vi "get_price.vi"(8 "error in (no error)":errorcluster, 11 "Furniture in":refnum<class "Furniture.lvclass">) -> (0 "error out":errorcluster, 2 "price":dbl, 3 "Furniture out":refnum<class "Furniture.lvclass">)   [LabVIEW 2024, in "Furniture.lvclass"]
uses:
  Furniture.lvclass
  Furniture.lvclass/Furniture.ctl
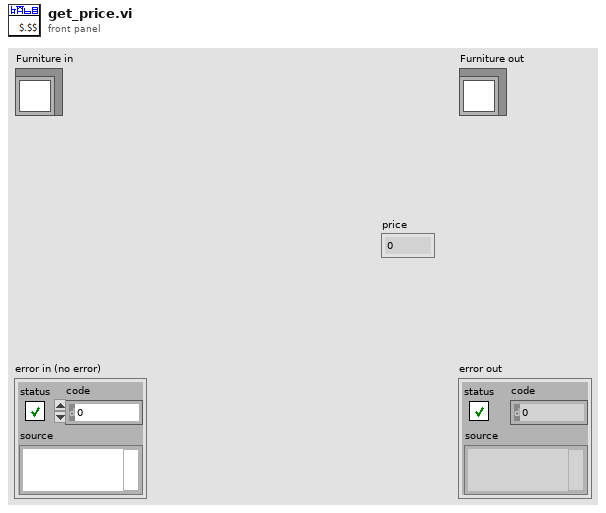
[diagram p1: front panel]
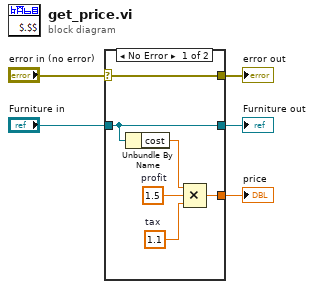
[diagram p0: block diagram]
diagram:
  n1 = case shown="No Error" "error in (no error)" {
    selector: "error in (no error)" -> [w11 w13]
    tunnel: [w11 w13] -> w4
    tunnel: [w10 w12] -> w2
    tunnel: "Furniture in" -> [w10 w12]
    tunnel: [w6 _] -> w1
    frame No Error {
      w7 = 1.1  # tax
      w8 = 1.5  # profit
      n2 = Unbundle By Name(w10) -> ("cost"=w9:dbl)
      n3 = Compound Arithmetic op=MULTIPLY(w9, w8, w7) -> (w6:dbl)
    }
    frame Error {
    }
  }
  "error out" <- w4
  "Furniture out" <- w2
  "price" <- w1
